vi "Protocol.vi"(8 "error in (no error)":errorcluster, 11 "Node Ptr":T1 format="%.0x") -> (0 "error out":errorcluster)   [LabVIEW 2020, in "Ballard MIL-STD-1553 System Explorer.lvlib" / "Implementation.lvlib"]
uses:
  Implementation.lvlib
  <vilib>/NI VeriStand/Custom Device API/Custom Device Item Ref.ctl
  <vilib>/NI VeriStand/Custom Device API/Custom Device API.lvlib
panel:
  in  "SHDocVw.IWebBrowser":refnum<k7>(container)
  in  "Specific Header":cluster{"Section Name":string}={"Section Name"="Specific Page Settings"}
  in  "General Header":cluster{"Section Name":string}={"Section Name"="General Page Settings"}
  in  "Description":string
  in  "Name":string
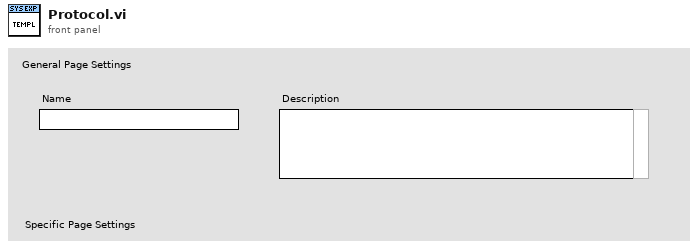
[diagram p1: front panel]
types:
  T1 = typedef "Custom Device API.lvlib/Custom Device Item Ref.ctl" = u64
  T2 = typedef "Custom Device API.lvlib/Custom Device Item Info.ctl" = cluster{"Name":string, "Is Channel":bool, "GUID":string, "Is Waveform":bool}
  T3 = typedef "Custom Device API.lvlib/Custom Device Commands.ctl" = enum16{"Default", "Item renamed", "Shutdown", "Dynamic button pressed"}
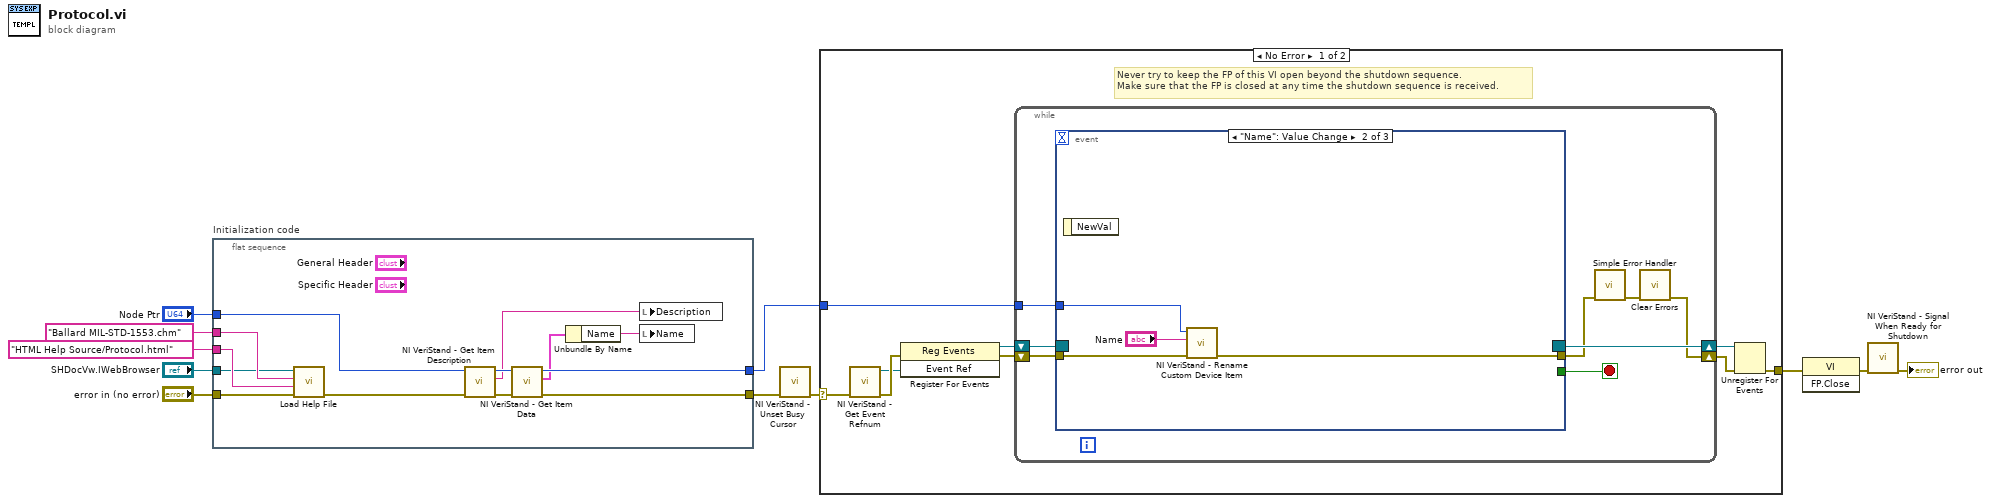
[diagram p0: block diagram]
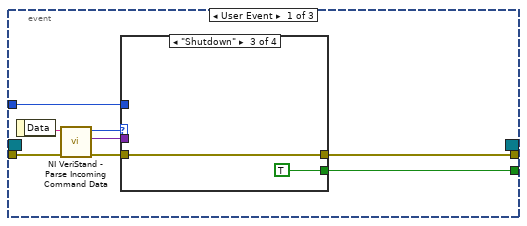
[diagram p2: hidden frame]
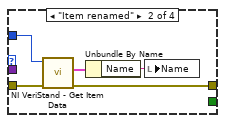
[diagram p4: hidden frame]
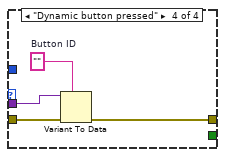
[diagram p5: hidden frame]
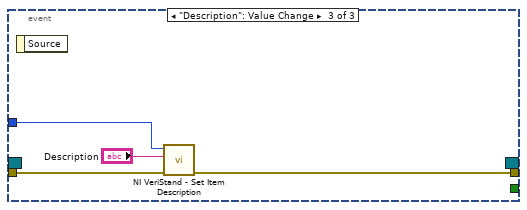
[diagram p6: hidden frame]
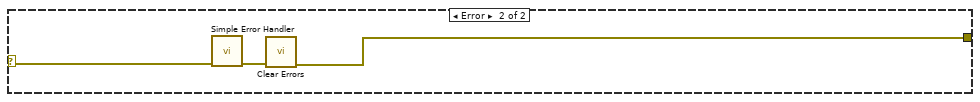
[diagram p7: hidden frame]
diagram:
  n1 = flat-sequence "Initialization code" {
    tunnel: "error in (no error)" -> [w16]
    tunnel: "Node Ptr" -> [w19]
    tunnel: [w20] -> w7
    tunnel: [w24] -> w4
    tunnel: "SHDocVw.IWebBrowser" -> [w12]
    tunnel: "HTML Help Source/Protocol.html" ("CD_CHM_Section") -> [w14]
    tunnel: "Ballard MIL-STD-1553.chm" ("CD_CHM_FileName") -> [w13]
    frame #0 {
      n2 = call "Load Help File.vi"("error in (no error)"=w16, "HTML File to Load"=w14, "Main CHM File"=w13, "Browser"=w12) -> ("error out"=w15:errorcluster)  [unwired: 7 in]
      n3 = call <vilib>:"NI VeriStand - Get Item Description.vi"("error in (no error)"=w15, "Item Ref in"=w19) -> ("error out"=w22:errorcluster, "Description"=w17:string, "Item Ref out"=w23:T1)  [unwired: 7 out]
      n4 = call <vilib>:"NI VeriStand - Get Item Data.vi"("error in (no error)"=w22, "Item Ref in"=w23) -> ("error out"=w20:errorcluster, "Item Info"=w21:T2, "Item Ref out"=w24:T1)  [unwired: 7 out]
      n5 = Unbundle By Name(w21) -> ("Name"=w18:string)
      n6 = local write "Description"(w17) -> ()
      n7 = local write "Name"(w18) -> ()
    }
  }
  n8 = call <vilib>:"NI VeriStand - Unset Busy Cursor.vi"("error in (no error)"=w7) -> ("error out"=w6:errorcluster)  [unwired: 10 out]
  n9 = case shown="No Error" w6 {
    selector: w6 -> [w25 w72]
    tunnel: [w30 w70] -> w11
    tunnel: w4 -> [w26 _]
    frame No Error {
      # "Never try to keep the FP of this VI open beyond the shutdown sequence.\nMake sure that the FP is closed at any time the shutdown sequence is received."
      n10 = call <vilib>:"NI VeriStand - Get Event Refnum.vi"("error in (no error)"=w25) -> ("error out"=w33:errorcluster, "Event Ref"=w29:refnum<user-event>)  [unwired: 9 out]
      n11 = register-events(error in=w33, w29) -> (reference out=w27:refnum<event-registration>, error out=w28:errorcluster)  [unwired: 1 in]
      n12 = while {
        tunnel: w26 -> [w37]
        shift-right: [w34] -> w31
        shift-left: w28 -> [w40]
        shift-right: [w41] -> w32
        shift-left: w27 -> [w39]
        stop <- w38 stop-if-true
        n13 = event shown="[1] \"Name\": Value Change" {
          selector: w39 -> [_ _ _]
          dyn-events: [_ _ _] -> w41
          timeout: _ -> [_ _ _]
          tunnel: w40 -> [w49 w65 w68]
          tunnel: [w45 _ _] -> w38
          tunnel: [w44 w64 w67] -> w36
          tunnel: w37 -> [w43 w63 w69]
          event User Event {
            n14 = event-data() -> ("Data"=w48:string)  [unwired: 1 out]
            n15 = call <vilib>:"NI VeriStand - Parse Incoming Command Data.vi"("error in (no error)"=w49, "Incoming data"=w48) -> ("error out"=w47:errorcluster, "Outgoing data"=w42:variant, "Action"=w46:T3)  [unwired: 7 out]
            n16 = case shown="\"Shutdown\"" w46 {
              tunnel: w47 -> [w50 w55 w56 w61]
              tunnel: [_ _ TRUE _] -> w45
              tunnel: [w50 w52 w56 w58] -> w44
              tunnel: w43 -> [_ w54 _ _]
              tunnel: w42 -> [_ _ _ w60]
              frame "Default", Default {
              }
              frame "Item renamed" {
                n17 = call <vilib>:"NI VeriStand - Get Item Data.vi"("error in (no error)"=w55, "Item Ref in"=w54) -> ("error out"=w52:errorcluster, "Item Info"=w53:T2)  [unwired: 8 out]
                n18 = Unbundle By Name(w53) -> ("Name"=w51:string)
                n19 = local write "Name"(w51) -> ()
              }
              frame "Shutdown" {
              }
              frame "Dynamic button pressed" {
                w59 = ""  # Button ID
                n20 = Variant To Data(error in=w61, type=w59, Variant=w60) -> (error out=w58:errorcluster)  [unwired: 1 out]
              }
            }
          }
          event "Name": Value Change {
            n21 = event-data() -> ()  [unwired: 2 out]
            n22 = call <vilib>:"NI VeriStand - Rename Custom Device Item.vi"("error in (no error)"=w65, "New Name"="Name", "Item Ref in"=w63) -> ("error out"=w64:errorcluster)  [unwired: 1 in, 7 out]
          }
          event "Description": Value Change {
            n23 = event-data() -> ()  [unwired: 2 out]
            n24 = call <vilib>:"NI VeriStand - Set Item Description.vi"("error in (no error)"=w68, "Description"="Description", "Item Ref in"=w69) -> ("error out"=w67:errorcluster)  [unwired: 8 out]
          }
        }
        n25 = call <vilib>:"Simple Error Handler.vi"("error in (no error)"=w36) -> ("error out"=w35:errorcluster)  [unwired: 1 in, 7 out]
        n26 = call <vilib>:"Clear Errors.vi"("error in (no error)"=w35) -> ("error out"=w34:errorcluster)  [unwired: 1 in, 5 out]
      }
      n27 = Unregister For Events(event registration refnum=w32, error in=w31) -> (error out=w30:errorcluster)
    }
    frame Error {
      n28 = call <vilib>:"Simple Error Handler.vi"("error in (no error)"=w72) -> ("error out"=w71:errorcluster)  [unwired: 1 in, 7 out]
      n29 = call <vilib>:"Clear Errors.vi"("error in (no error)"=w71) -> ("error out"=w70:errorcluster)  [unwired: 1 in, 5 out]
    }
  }
  n30 = invoke class="VI" method="FP.Close"(error in=w11) -> (error out=w10:errorcluster)  [unwired: 2 in, 2 out]
  n31 = call <vilib>:"NI VeriStand - Signal When Ready for Shutdown.vi"("error in (no error)"=w10) -> ("error out"=→"error out":errorcluster)  [unwired: 10 out]
